vi "LHF.DB.Mongo.Client.Disconnect.vi"(8 "error in (no error)":errorcluster, 11 "LHF.DB.Mongo in":refnum<class "LHF.DB.Mongo.lvclass">) -> (0 "error out":errorcluster, 3 "LHF.DB.Mongo out":refnum<class "LHF.DB.Mongo.lvclass">)   [LabVIEW 2013, in "LHF.DB.Mongo.lvclass"]
uses:
  LHF.DB.Mongo.lvclass
  LHF.DB.Mongo.lvclass/LHF.DB.Mongo.ctl
  C:/Users/schim/Desktop/Projetos/LabVIEW-MongoDB/src/Driver/MongoDB.Driver.dll
  Driver/MongoDB.Driver.dll
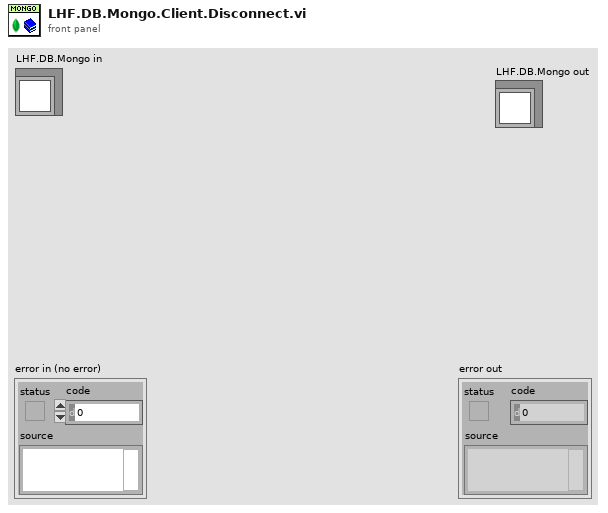
[diagram p1: front panel]
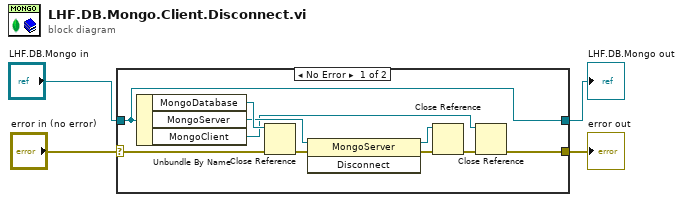
[diagram p0: block diagram]
diagram:
  n1 = case shown="No Error" "error in (no error)" {
    selector: "error in (no error)" -> [w7 w16]
    tunnel: [w6 w16] -> w3
    tunnel: [w5 w15] -> w1
    tunnel: "LHF.DB.Mongo in" -> [w5 w15]
    frame No Error {
      n2 = Unbundle By Name(w5) -> ("MongoDatabase"=w13:refnum<k24>, "MongoServer"=w12:refnum<k24>, "MongoClient"=w11:refnum<k24>)
      n3 = Close Reference(reference=w13, error in (no error)=w7) -> (error out=w9:errorcluster)
      n4 = invoke class="MongoServer" method="Disconnect"(reference=w12, error in=w9) -> (reference out=w10:refnum<k24>, error out=w8:errorcluster)  [unwired: 1 in, 1 out]
      n5 = Close Reference(reference=w10, error in (no error)=w8) -> (error out=w14:errorcluster)
      n6 = Close Reference(reference=w11, error in (no error)=w14) -> (error out=w6:errorcluster)
    }
    frame Error {
    }
  }
  "error out" <- w3
  "LHF.DB.Mongo out" <- w1
